vi "Initialize FIU References.vi"(8 "error in (no error)":errorcluster, 10 "FIU Engine Data in":T8 {"Ordered Fault Channels" format="%.0x"; "FIU IDs"."Slot #" max=15; "FIU IDs"."Chip Address (A2 A1 A0)" max=7}, 11 "Device Ref in":T7=18446744073709551615 format="%.0x") -> (0 "error out":errorcluster, 2 "FIU Engine Refs":T1 {"FIU IDs"."Slot #" max=15; "FIU IDs"."Chip Address (A2 A1 A0)" max=7; "FIU Block Data Refs"."Data Reference" format="%.0x"}, 3 "Device Ref out":T7=18446744073709551615 format="%.0x")   [LabVIEW 2014, in "SLSC configuration Engine.lvlib"]
uses:
  SLSC configuration Engine.lvlib
  Shared/Type Defs/FIU Engine Data.ctl
  Shared/Type Defs/FIU IDs.ctl
  Example/SPI Utility/Slot #.ctl
  Example/MCP23S17/Chip Address.ctl
  <vilib>/NI Veristand/Custom Device API/Custom Device Item Ref.ctl
  Type Defs/FIU Engine Refs.ctl
  <vilib>/NI Veristand/Custom Device API/Block Data Reference.ctl
  <vilib>/NI Veristand/Custom Device API/Data Reference.ctl
  <vilib>/NI Veristand/Custom Device API/Data Access Type.ctl
  <vilib>/NI Veristand/Custom Device API/Custom Device API.lvlib
  Shared/SLSC configuration Shared.lvlib
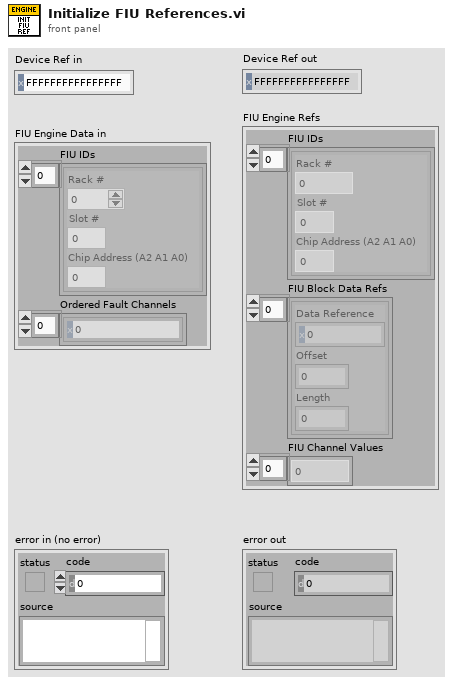
[diagram p1: front panel]
types:
  T1 = typedef "SLSC configuration Engine.lvlib/FIU Engine Refs.ctl" = cluster{"FIU IDs":T2[], "FIU Block Data Refs":T5[], "FIU Channel Values":dbl[]}
  T2 = typedef "SLSC configuration Shared.lvlib/FIU IDs.ctl" = cluster{"Rack #":u8, "Slot #":T3, "Chip Address (A2 A1 A0)":T4}
  T3 = typedef "SLSC configuration Shared.lvlib/Slot #.ctl" = u8
  T4 = typedef "SLSC configuration Shared.lvlib/Chip Address.ctl" = u8
  T5 = typedef "Custom Device API.lvlib/Block Data Reference.ctl" = cluster{"Data Reference":T6, "Offset":i32, "Length":i32}
  T6 = typedef "Custom Device API.lvlib/Data Reference.ctl" = i32
  T7 = typedef "Custom Device API.lvlib/Custom Device Item Ref.ctl" = u64
  T8 = typedef "SLSC configuration Shared.lvlib/FIU Engine Data.ctl" = cluster{"FIU IDs":T2[], "Ordered Fault Channels":T7[]}
  T9 = typedef "Custom Device API.lvlib/Data Access Type.ctl" = enum16{"Read", "Write"}
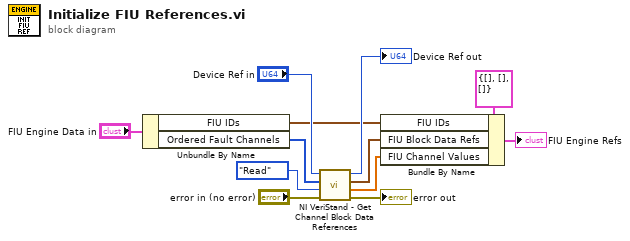
[diagram p0: block diagram]
diagram:
  n1 = Unbundle By Name("FIU Engine Data in") -> ("FIU IDs"=w4:T2[], "Ordered Fault Channels"=w11:T7[])
  n2 = call <vilib>:"NI VeriStand - Get Channel Block Data References.vi"("error in (no error)"="error in (no error)", "Access"=Data_Access_Type."Read", "Channel Refs"=w11, "Device Ref in"="Device Ref in") -> ("error out"=→"error out":errorcluster, "Values Array"=w2:dbl[], "Block Data Refs"=w3:T5[], "Device Ref out"=→"Device Ref out":T7)  [unwired: 4 in]
  n3 = Bundle By Name(cluster=T1 {"FIU IDs"=[], "FIU Block Data Refs"=[], "FIU Channel Values"=[]}, "FIU IDs"=w4, "FIU Block Data Refs"=w3, "FIU Channel Values"=w2) -> (→"FIU Engine Refs":T1)
